vi "1D I64 To String with Under Line.vi"(10 "Array In":i64[](array[numeric])) -> (2 "String out":string)   [LabVIEW 2019]
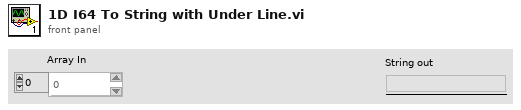
[diagram p1: front panel]
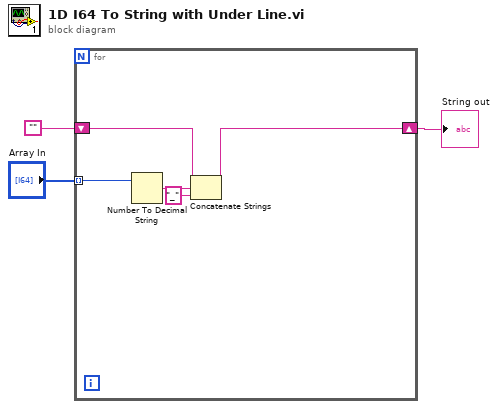
[diagram p0: block diagram]
diagram:
  n1 = for {
    tunnel: "Array In" -> [w8] mode=indexing
    shift-right: [w4] -> w1
    shift-left: "" -> [w5]
    n2 = Number To Decimal String(number=w8) -> (decimal integer string=w7:string)  [unwired: 1 in]
    n3 = Concatenate Strings(w5, w7, "_" ("string")) -> (w4:string)
  }
  "String out" <- w1
